vi "update_MagFieldTable.vi"(8 "error in (no error)":errorcluster, 9 "new magnet value":string, 10 "isotope name":string, 11 "MFT name":string) -> (0 "error out":errorcluster)   [LabVIEW 2018]
doc: "updates the MagFieldTableObject (given by MFT name)\nwith a new magnet value for the isotope (give by isotope name)\n\nIt also updates the MagFieldTables.ini with the most recent data."
uses:
  Classes/MagFieldTable/MagFieldTable.lvclass
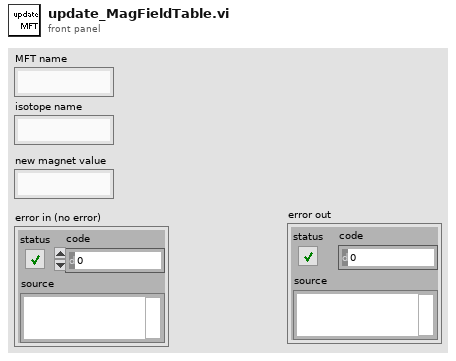
[diagram p1: front panel]
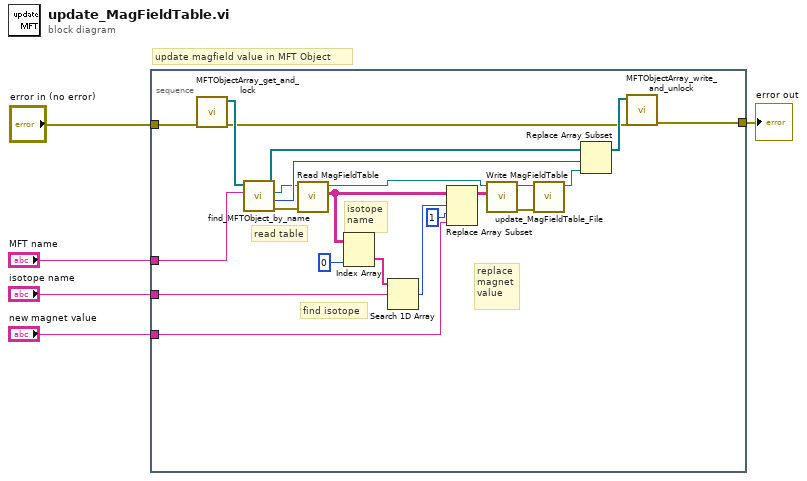
[diagram p0: block diagram]
diagram:
  # "update magfield value in MFT Object"
  n1 = stacked-sequence {
    tunnel: "new magnet value" -> [w9]
    tunnel: "isotope name" -> [w10]
    tunnel: "MFT name" -> [w11]
    tunnel: "error in (no error)" -> [w14]
    tunnel: [w12] -> w1
    frame #0 {
      # "isotope\nname"
      # "read table"
      # "replace\nmagnet\nvalue"
      # "find isotope"
      n2 = call "MFTObjectArray_get_and_lock.vi"("error in (no error)"=w14) -> ("error out"=w13:errorcluster, "MFTObjects"=w22:refnum<class "MagFieldTable.lvclass">[])  [unwired: 9 in]
      n3 = call "find_MFTObject_by_name.vi"("MFT name"=w11, "MFTObjects in"=w22) -> ("error out"=w18:errorcluster, "index of found"=w25:i32, "found AnalyisObject"=w17:refnum<class "MagFieldTable.lvclass">, "MFTObjects out"=w24:refnum<class "MagFieldTable.lvclass">[])  [unwired: 6 in]
      n4 = call-dynamic "Read MagFieldTable.vi"("error in (no error)"=w18, "MagFieldTable in"=w17) -> ("MagFieldTable"=w19:string[][], "MagFieldTable out"=w27:refnum<class "MagFieldTable.lvclass">)  [unwired: 7 in, 1 out]
      n5 = Index Array(array=w19, index (col)=0 ("disabled index (col)")) -> (element=w15:string[])  [unwired: 1 in]
      n6 = Search 1D Array(1D array=w15, element=w10) -> (index of element=w20:i32)  [unwired: 1 in]
      n7 = Replace Array Subset(array=w19, new element=w9, index (row)=w20, index (col)=1 ("disabled index (col)")) -> (w26:string[][])
      n8 = call-dynamic "Write MagFieldTable.vi"("MagFieldTable"=w26, "MagFieldTable in"=w27) -> ("error out"=w7:errorcluster, "MagFieldTable out"=w8:refnum<class "MagFieldTable.lvclass">)  [unwired: 8 in]
      n9 = call "update_MagFieldTable_File.vi"("error in (no error)"=w7, "MFTObj in"=w8) -> ("MFTObj out"=w6:refnum<class "MagFieldTable.lvclass">)  [unwired: 8 in, 1 out]
      n10 = Replace Array Subset(array=w24, new element=w6, index=w25) -> (w23:refnum<class "MagFieldTable.lvclass">[])
      n11 = call "MFTObjectArray_write_and_unlock.vi"("error in (no error)"=w13, "MFTObjects"=w23) -> ("error out"=w12:errorcluster)  [unwired: 9 in]
    }
  }
  "error out" <- w1
